vi "Generate Param Config XML.vi"() -> ()   [LabVIEW 2017]
panel:
  in  "Rx Start Channel":i32
  in  "Tx Start Channel":i32
  in  "Tx start bit":i32=10
  in  "Tx number of bits":i32=16
  in  "Rx number of bits":i32=16
  in  "Rx start bit":i32=10
  in  "file path (use dialog)":path
  in  "Number of Tx Channels":i32
  in  "Labels per Tx Channel":i32
  in  "Number of Rx Channels":i32
  in  "Labels per Rx Channel":i32
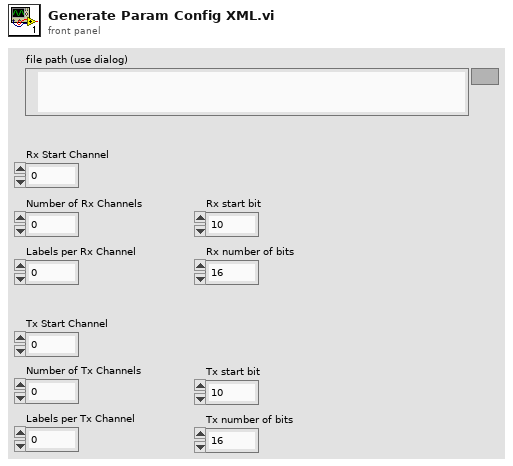
[diagram p1: front panel]
types:
  T1 = enum16{"open", "replace", "create", "open or create", "replace or create", "replace or create with confirmation"}
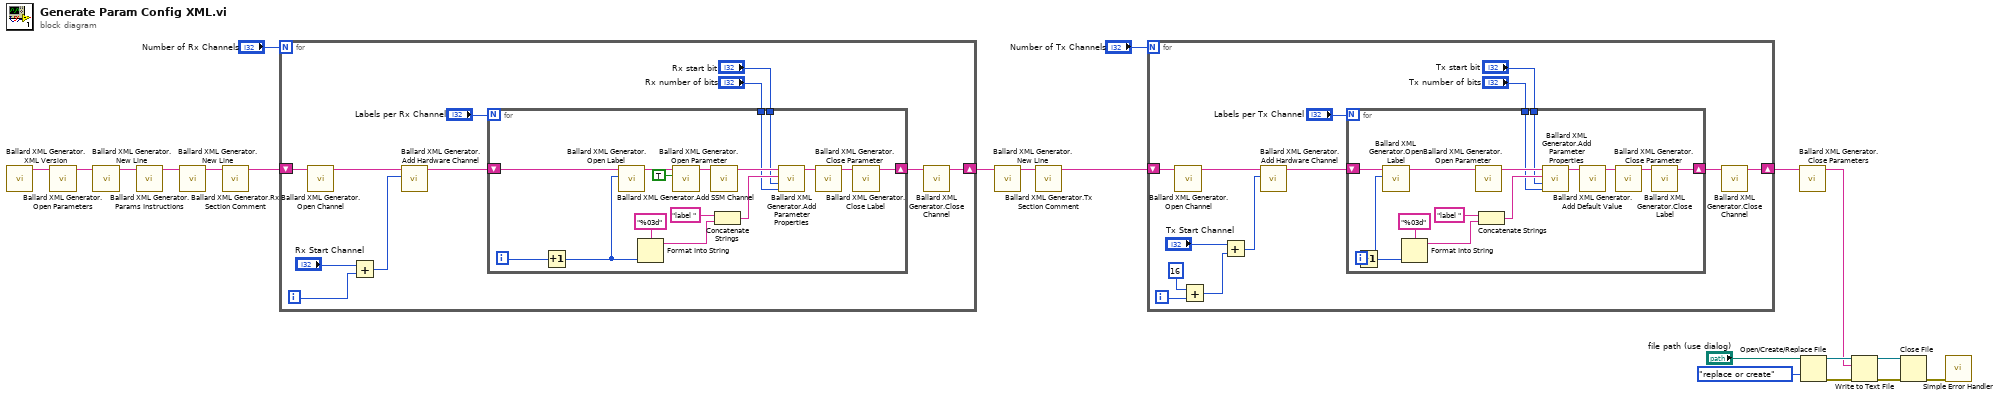
[diagram p0: block diagram]
diagram:
  n1 = call "Ballard XML Generator.XML Version.vi"() -> ("string out"=w12:string)  [unwired: 11 in]
  n2 = call "Ballard XML Generator.Open Parameters.vi"("string in"=w12) -> ("string out"=w11:string)  [unwired: 10 in]
  n3 = call "Ballard XML Generator.New Line.vi"("string in"=w11) -> ("string out"=w10:string)  [unwired: 10 in]
  n4 = call "Ballard XML Generator.Params Instructions.vi"("string in"=w10) -> ("string out"=w9:string)  [unwired: 10 in]
  n5 = call "Ballard XML Generator.New Line.vi"("string in"=w9) -> ("string out"=w8:string)  [unwired: 10 in]
  n6 = call "Ballard XML Generator.Rx Section Comment.vi"("string in"=w8) -> ("string out"=w6:string)  [unwired: 10 in]
  n7 = for {
    N: "Number of Rx Channels" -> [_]
    shift-right: [w24] -> w5
    shift-left: w6 -> [w29]
    i -> [w22]
    n8 = call "Ballard XML Generator.Open Channel.vi"("string in"=w29) -> ("string out"=w30:string)  [unwired: 10 in]
    n9 = Add(x="Rx Start Channel", y=w22) -> (x+y=w21:i32)
    n10 = call "Ballard XML Generator.Add Hardware Channel.vi"("channel"=w21, "string in"=w30) -> ("string out"=w28:string)  [unwired: 9 in]
    n11 = for {
      N: "Labels per Rx Channel" -> [_]
      shift-right: [w41] -> w25
      shift-left: w28 -> [w44]
      tunnel: "Rx start bit" -> [w36]
      tunnel: "Rx number of bits" -> [w35]
      i -> [w33]
      n12 = Increment(x=w33) -> (x+1=w32:i32)
      n13 = call "Ballard XML Generator.Open Label.vi"("label decimal"=w32, "string in"=w44) -> ("string out"=w45:string)  [unwired: 9 in]
      n14 = Format Into String(format string="%03d", w32) -> (resulting string=w40:string)  [unwired: 2 in, 1 out]
      n15 = call "Ballard XML Generator.Add SSM Channel.vi"("create SSM chan?"=TRUE, "string in"=w45) -> ("string out"=w46:string)  [unwired: 9 in]
      n16 = call "Ballard XML Generator.Open Parameter.vi"("string in"=w46) -> ("string out"=w47:string)  [unwired: 10 in]
      n17 = Concatenate Strings("label ", w40) -> (w37:string)
      n18 = call "Ballard XML Generator.Add Parameter Properties.vi"("number of bits"=w35, "start bit"=w36, "name"=w37, "string in"=w47) -> ("string out"=w34:string)  [unwired: 7 in]
      n19 = call "Ballard XML Generator.Close Parameter.vi"("string in"=w34) -> ("string out"=w42:string)  [unwired: 10 in]
      n20 = call "Ballard XML Generator.Close Label.vi"("string in"=w42) -> ("string out"=w41:string)  [unwired: 10 in]
    }
    n21 = call "Ballard XML Generator.Close Channel.vi"("string in"=w25) -> ("string out"=w24:string)  [unwired: 10 in]
  }
  n22 = call "Ballard XML Generator.New Line.vi"("string in"=w5) -> ("string out"=w7:string)  [unwired: 10 in]
  n23 = call "Ballard XML Generator.Tx Section Comment.vi"("string in"=w7) -> ("string out"=w2:string)  [unwired: 10 in]
  n24 = for {
    N: "Number of Tx Channels" -> [_]
    shift-right: [w54] -> w1
    shift-left: w2 -> [w59]
    i -> [w52]
    n25 = call "Ballard XML Generator.Open Channel.vi"("string in"=w59) -> ("string out"=w60:string)  [unwired: 10 in]
    n26 = Add(x=16, y=w52) -> (x+y=w49:i32)
    n27 = Add(x="Tx Start Channel", y=w49) -> (x+y=w48:i32)
    n28 = call "Ballard XML Generator.Add Hardware Channel.vi"("channel"=w48, "string in"=w60) -> ("string out"=w58:string)  [unwired: 9 in]
    n29 = for {
      N: "Labels per Tx Channel" -> [_]
      shift-right: [w72] -> w55
      shift-left: w58 -> [w74]
      tunnel: "Tx start bit" -> [w67]
      tunnel: "Tx number of bits" -> [w66]
      i -> [w62]
      n30 = Increment(x=w62) -> (x+1=w61:i32)
      n31 = call "Ballard XML Generator.Open Label.vi"("label decimal"=w61, "string in"=w74) -> ("string out"=w63:string)  [unwired: 9 in]
      n32 = Format Into String(format string="%03d", w61) -> (resulting string=w71:string)  [unwired: 2 in, 1 out]
      n33 = call "Ballard XML Generator.Open Parameter.vi"("string in"=w63) -> ("string out"=w75:string)  [unwired: 10 in]
      n34 = Concatenate Strings("label ", w71) -> (w68:string)
      n35 = call "Ballard XML Generator.Add Parameter Properties.vi"("number of bits"=w66, "start bit"=w67, "name"=w68, "string in"=w75) -> ("string out"=w65:string)  [unwired: 7 in]
      n36 = call "Ballard XML Generator.Add Default Value.vi"("string in"=w65) -> ("string out"=w64:string)  [unwired: 10 in]
      n37 = call "Ballard XML Generator.Close Parameter.vi"("string in"=w64) -> ("string out"=w73:string)  [unwired: 10 in]
      n38 = call "Ballard XML Generator.Close Label.vi"("string in"=w73) -> ("string out"=w72:string)  [unwired: 10 in]
    }
    n39 = call "Ballard XML Generator.Close Channel.vi"("string in"=w55) -> ("string out"=w54:string)  [unwired: 10 in]
  }
  n40 = call "Ballard XML Generator.Close Parameters.vi"("string in"=w1) -> ("string out"=w4:string)  [unwired: 10 in]
  n41 = Open/Create/Replace File(file path (use dialog)="file path (use dialog)", operation (0:open)=T1."replace or create") -> (refnum out=w17:refnum<file>, error out=w16:errorcluster)  [unwired: 4 in, 1 out]
  n42 = Write to Text File(file (use dialog)=w17, text=w4, error in=w16) -> (refnum out=w15:refnum<file>, error out=w14:errorcluster)  [unwired: 1 in, 1 out]
  n43 = Close File(refnum=w15, error in=w14) -> (error out=w13:errorcluster)  [unwired: 1 out]
  n44 = call <vilib>:"Simple Error Handler.vi"("error in (no error)"=w13) -> ()  [unwired: 4 in, 5 out]
